vi "ConstantToArray_U32Rgba.vi"(11 "Constant":T1) -> (3 "ConstantArray":dbl[](array[numeric]))   [LabVIEW 2020, in "OpenLvVision_OpenCv.lvlib"]
uses:
  OpenLvVision_OpenCv.lvlib
  <vilib>/OpenLvVision/OpenLvVision_Image/DataAccess/TypeDef/OLV RgbaU32.ctl
  <vilib>/OpenLvVision/OpenLvVision_Image/DataAccess/OLV DataAccess.lvlib
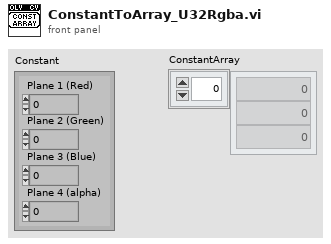
[diagram p1: front panel]
types:
  T1 = typedef "OLV OpenLvVision_Image.lvlib/OLV DataAccess.lvlib/OLV RgbaU32.ctl" = cluster{"Plane 1 (Red)":u8, "Plane 2 (Green)":u8, "Plane 3 (Blue)":u8, "Plane 4 (alpha)":u8}
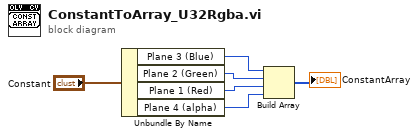
[diagram p0: block diagram]
diagram:
  n1 = Unbundle By Name("Constant") -> ("Plane 3 (Blue)"=w6:u8, "Plane 2 (Green)"=w5:u8, "Plane 1 (Red)"=w4:u8, "Plane 4 (alpha)"=w3:u8)
  n2 = Build Array(w6, w5, w4, w3) -> (→"ConstantArray":u8[])
